vi "boot.vi"(8 "error in (no error)":errorcluster, 10 "Model in":refnum<class "Model.lvclass">, 11 "InitialState in":refnum<class "InitialState.lvclass">) -> (0 "error out":errorcluster, 2 "Model out":refnum<class "Model.lvclass">, 3 "InitialState out":refnum<class "InitialState.lvclass">)   [LabVIEW 2016, in "InitialState.lvclass"]
uses:
  InitialState.lvclass
  Model/Model.lvclass
  DataTypes/Topics/Parts/DetailedStates.ctl
  Model/Model.lvclass/Model.ctl
  Publisher/Publisher.lvclass/Publisher.ctl
  Communicator/M1M3SAL/M1M3SAL.lvclass/M1M3SAL.ctl
  Publisher/transmit.vi
  Communicator/M1M3SAL/transmit.vi
  Communicator/M1M3SAL/write.vi
  Model/populateEventSummaryState.vi
  Model/publishEventSummaryState.vi
  Model/populateEventDetailedState.vi
  Model/publishEventDetailedState.vi
  DataTypes/Topics/M1M3SupportTopics.lvlib
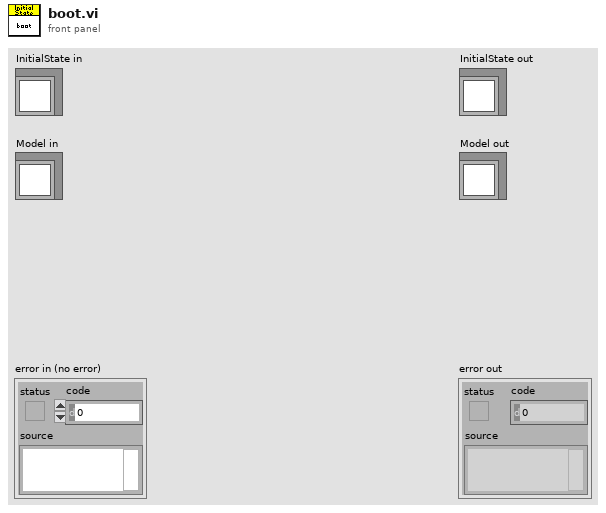
[diagram p1: front panel]
types:
  T1 = typedef "M1M3SupportTopics.lvlib/DetailedStates.ctl" = enum16{"OfflineState", "InitialState", "StandbyState", "DisabledState", "ParkedState", "FaultState", "ParkedMaintenanceState", "ActiveMaintenanceState"}
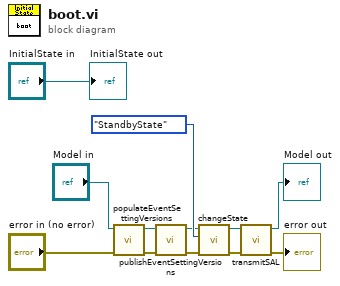
[diagram p0: block diagram]
diagram:
  n1 = call "populateEventSettingVersions.vi"("error in (no error)"="error in (no error)", "Model in"="Model in") -> ("error out"=w6:errorcluster, "Model out"=w9:refnum<class "Model.lvclass">)  [unwired: 8 in]
  n2 = call "publishEventSettingVersions.vi"("error in (no error)"=w6, "Model in"=w9) -> ("error out"=w5:errorcluster, "Model out"=w8:refnum<class "Model.lvclass">)  [unwired: 8 in]
  n3 = call "changeState.vi"("error in (no error)"=w5, "DetailedStates"=DetailedStates."StandbyState", "Model in"=w8) -> ("error out"=w2:errorcluster, "Model out"=w4:refnum<class "Model.lvclass">)  [unwired: 7 in]
  n4 = call "transmitSAL.vi"("error in (no error)"=w2, "Model in"=w4) -> ("error out"=→"error out":errorcluster, "Model out"=→"Model out":refnum<class "Model.lvclass">)  [unwired: 8 in]
  "InitialState out" <- "InitialState in"
